vi "Pressure_DAQ_subvi.vi"(3 "Number of Samples":i32=1000) -> (0 "Waveform Chart":waveform(dbl)(graph), 7 "pressure_Vdc":dbl[](array[numeric]), 8 "density_constant":dbl[](array[numeric]), 9 "temp_constant":dbl[](array[numeric]), 10 "unix_time":dbl[](array[numeric]) format="%#_21g")   [LabVIEW 2023]
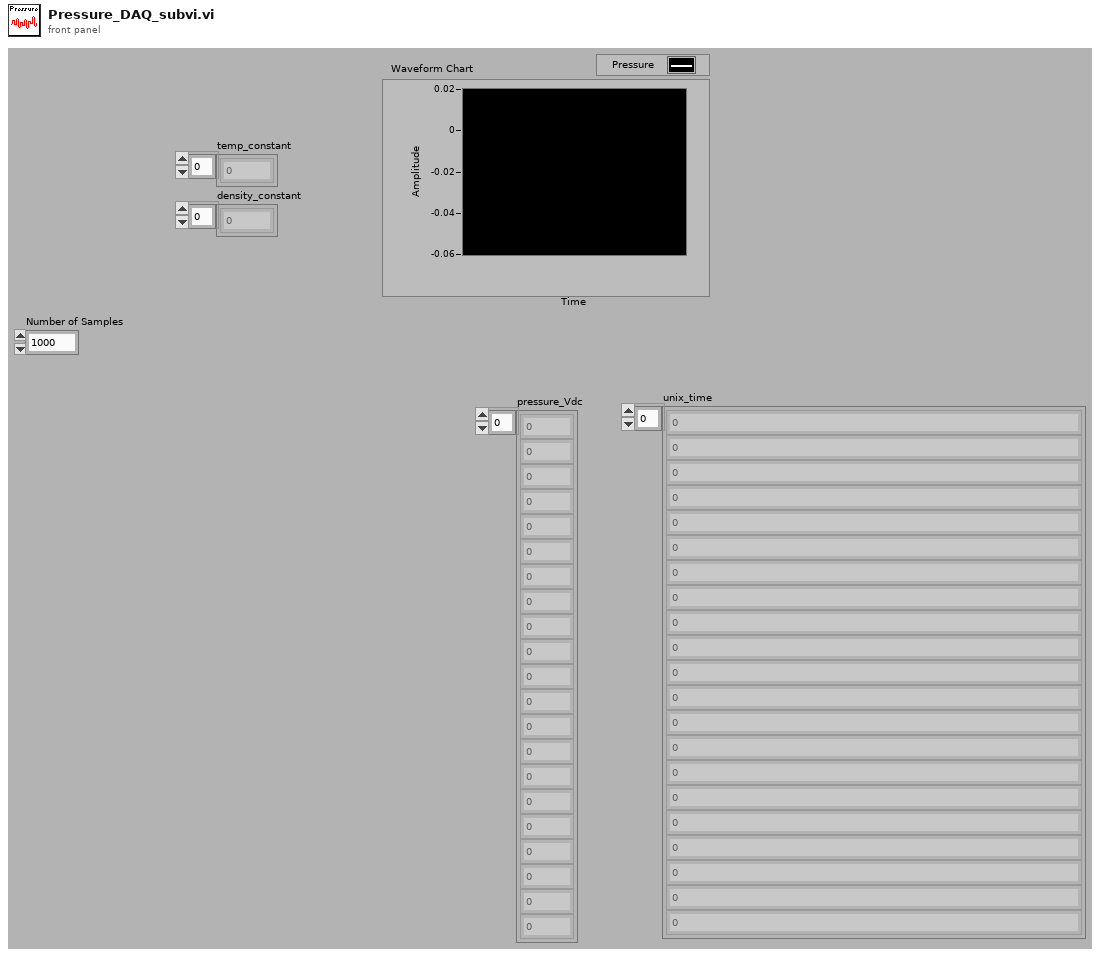
[diagram p1: front panel]
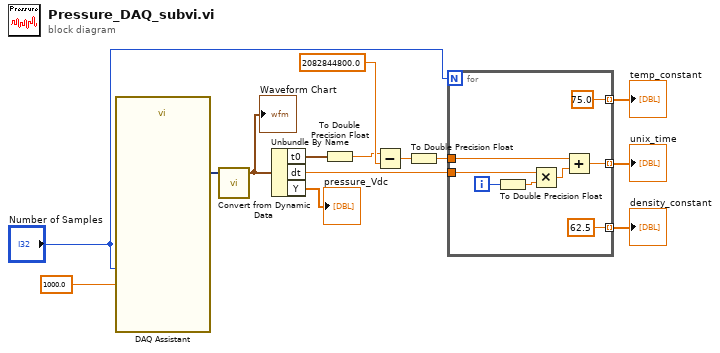
[diagram p0: block diagram]
diagram:
  n1 = call "DAQ Assistant"("rate"=1000.0 ("Sampling Rate"), "number of samples"="Number of Samples") -> ("data"=w12:dynamicdata)  [unwired: 14 in, 3 out]
  n2 = call "Convert from Dynamic Data"("Dynamic Data Type"=w12) -> ("Waveform"=w11:waveform(dbl))  [unwired: 3 in]
  "Waveform Chart" <- w11
  n3 = Unbundle By Name(w11) -> ("t0"=w8:timestamp, "dt"=w10:dbl, "Y"=→"pressure_Vdc":dbl[])
  n4 = To Double Precision Float(number=w8) -> (double precision float=w6:dbl)
  n5 = Subtract(x=w6, y=2082844800.0) -> (x-y=w9:dbl)
  n6 = To Double Precision Float(number=w9) -> (double precision float=w5:dbl)
  n7 = for {
    N: "Number of Samples" -> [_]
    tunnel: w10 -> [w21]
    tunnel: [75.0] -> w3 mode=indexing
    tunnel: [62.5] -> w2 mode=indexing
    tunnel: [w17] -> w4 mode=indexing
    tunnel: w5 -> [w16]
    i -> [w20]
    n8 = To Double Precision Float(number=w20) -> (double precision float=w15:dbl)
    n9 = Multiply(x=w21, y=w15) -> (x*y=w22:dbl)
    n10 = Add(x=w16, y=w22) -> (x+y=w17:dbl)
  }
  "unix_time" <- w4
  "temp_constant" <- w3
  "density_constant" <- w2
